vi "Simple Digital Input Example - Daniel Logic.vi"() -> ()   [LabVIEW 2011]
doc: "This example shows how to read values from a digital channel.\n\nIt will display the digital value as Low (LED off) or High (LED on).\n\nThis example works with the NI 9403 module connected to a Digital Sidecar. The Digital Sidecar should have 12V applied to the WAGO connector. Note that the digital channels are pulled high when floating. This means that if you want to read a limit switch, you would need to connect one end of the switch to SIG and the other end to (-). The the LED would be On when the switch is open and Off when the switch is closed."
uses:
  <vilib>/Rock Robotics/SystemInterfaces/DIO/FPGA_DIOChannel.ctl
  <vilib>/Rock Robotics/SystemInterfaces/Typedef/FPGA_TypedefDigitalModule.ctl
panel:
  out "Numeric":dbl
  out "Digital Input Value 4":bool
  in  "DIO Module 4":T1
  in  "DIO Channel 4":T2
  out "Digital Input Value 3":bool
  in  "DIO Module 3":T1
  in  "DIO Channel 3":T2
  out "Digital Input Value 2":bool
  in  "DIO Channel 2":T2
  in  "DIO Module 2":T1
  in  "DIO Module":T1
  out "Digital Input Value":bool
  in  "DIO Channel":T2
  in  "stop":bool
  # "Wiring Diagram for Digital Sidecar connected to an NI 9403"
  # "Set these inputs before running."
  # "PWR"
  # "SIG"
  # "(-)"
  # "14\n13\n12\n11\n10\n9\n8\n7\n6\n5\n4\n3\n2\n1"
  # "DIGITAL I/O"
  # "TTL Signal"
  # "This shows wiring for a TTL signal.  To read a switch, wire one side of the switch to SIG and the other side to (-).  The LED will be On when the switch is open and Off when the switch is closed."
  # "Digital Sidecar"
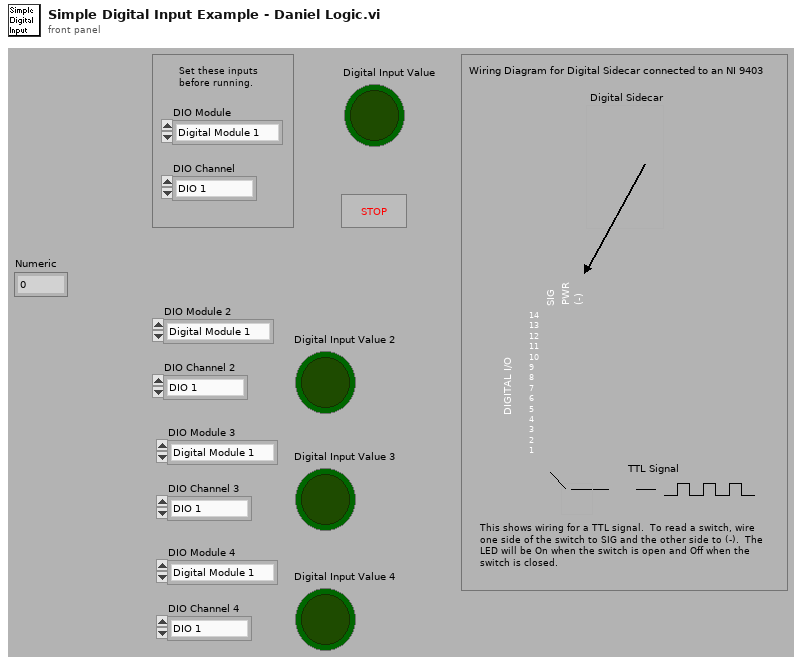
[diagram p1: front panel]
types:
  T1 = typedef "FPGA_TypedefDigitalModule.ctl" = enum16{"Digital Module 1", "Digital Module 2"}
  T2 = typedef "FPGA_DIOChannel.ctl" = enum8{"DIO 1", "DIO 2", "DIO 3", "DIO 4", "DIO 5", "DIO 6", "DIO 7", "DIO 8", "DIO 9", "DIO 10", "DIO 11", "DIO 12", "DIO 13", "DIO 14", "Invalid"}
  T3 = typedef "WPI_DigitalInputDevRef.ctl" = cluster{"DevStatus":errorcluster, "DIO Channel":T2, "Digital Module":T1}
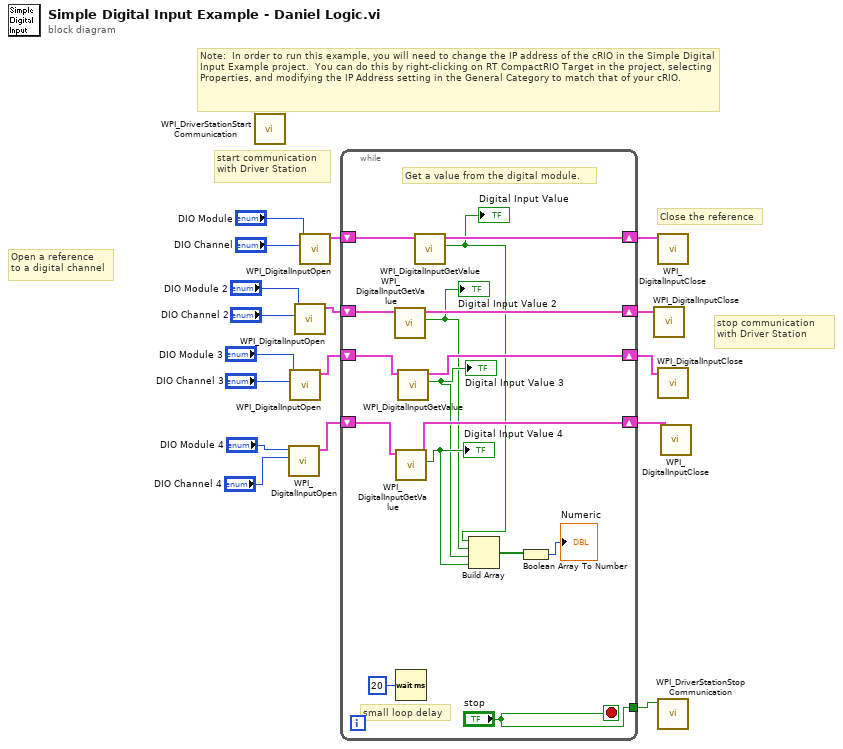
[diagram p0: block diagram]
diagram:
  # "stop communication with Driver Station"
  # "start communication with Driver Station"
  # "Note:  In order to run this example, you will need to change the IP address of the cRIO in the Simple Digital Input Example project.  You can do this by right-clicking on RT CompactRIO Target in the project, selecting Properties, and modifying the IP Address setting in the General Category to match that of your cRIO."
  # "Close the reference"
  # "Open a reference\nto a digital channel"
  n1 = call <vilib>:"WPI_DriverStationStart Communication.vi"() -> ()  [unwired: 1 in, 11 out]
  n2 = call <vilib>:"WPI_DigitalInputOpen.vi"("DIO Channel"="DIO Channel 4", "Digital Module (Module 1)"="DIO Module 4") -> ("DigitalInputDevRef"=w2:T3)  [unwired: 1 in, 8 out]
  n3 = call <vilib>:"WPI_DigitalInputOpen.vi"("DIO Channel"="DIO Channel 3", "Digital Module (Module 1)"="DIO Module 3") -> ("DigitalInputDevRef"=w6:T3)  [unwired: 1 in, 8 out]
  n4 = call <vilib>:"WPI_DigitalInputOpen.vi"("DIO Channel"="DIO Channel 2", "Digital Module (Module 1)"="DIO Module 2") -> ("DigitalInputDevRef"=w10:T3)  [unwired: 1 in, 8 out]
  n5 = call <vilib>:"WPI_DigitalInputOpen.vi"("DIO Channel"="DIO Channel", "Digital Module (Module 1)"="DIO Module") -> ("DigitalInputDevRef"=w16:T3)  [unwired: 1 in, 8 out]
  n6 = while {
    shift-right: [w32] -> w15
    shift-left: w16 -> [w33]
    tunnel: ["stop"] -> w14
    shift-right: [w28] -> w9
    shift-left: w10 -> [w29]
    shift-right: [w26] -> w5
    shift-left: w6 -> [w27]
    shift-right: [w24] -> w1
    shift-left: w2 -> [w25]
    stop <- "stop" stop-if-true
    # "small loop delay"
    # "Get a value from the digital module."
    n7 = call <vilib>:"WPI_DigitalInputGetValue.vi"("DigitalInputDevRef"=w29) -> ("Value"=w21:bool, "DigitalInputDevRef"=w28:T3)  [unwired: 1 in, 8 out]
    "Digital Input Value 2" <- w21
    n8 = call <vilib>:"WPI_DigitalInputGetValue.vi"("DigitalInputDevRef"=w25) -> ("Value"=w23:bool, "DigitalInputDevRef"=w24:T3)  [unwired: 1 in, 8 out]
    "Digital Input Value 4" <- w23
    n9 = Wait (ms)(milliseconds to wait=u32 20) -> ()  [unwired: 1 out]
    n10 = call <vilib>:"WPI_DigitalInputGetValue.vi"("DigitalInputDevRef"=w27) -> ("Value"=w22:bool, "DigitalInputDevRef"=w26:T3)  [unwired: 1 in, 8 out]
    "Digital Input Value 3" <- w22
    n11 = call <vilib>:"WPI_DigitalInputGetValue.vi"("DigitalInputDevRef"=w33) -> ("Value"=w20:bool, "DigitalInputDevRef"=w32:T3)  [unwired: 1 in, 8 out]
    "Digital Input Value" <- w20
    n12 = Build Array(w20, w21, w22, w23) -> (w19:bool[])
    n13 = Boolean Array To Number(Boolean array=w19) -> (number=→"Numeric":u32)
  }
  n14 = call <vilib>:"WPI_DigitalInputClose.vi"("DigitalInputDevRef"=w9) -> ()  [unwired: 1 in, 10 out]
  n15 = call <vilib>:"WPI_DigitalInputClose.vi"("DigitalInputDevRef"=w15) -> ()  [unwired: 1 in, 10 out]
  n16 = call <vilib>:"WPI_DigitalInputClose.vi"("DigitalInputDevRef"=w5) -> ()  [unwired: 1 in, 10 out]
  n17 = call <vilib>:"WPI_DriverStationStop Communication.vi"("StopCommunication"=w14) -> ()  [unwired: 1 in, 10 out]
  n18 = call <vilib>:"WPI_DigitalInputClose.vi"("DigitalInputDevRef"=w1) -> ()  [unwired: 1 in, 10 out]
